vi "visObs (SubVI).vi"(1 "obsts":cluster{"x prior ":i32, "y prior":i32}[](array[cluster])) -> (0 "invisObsts":T1(array[cluster]))   [LabVIEW 2011]
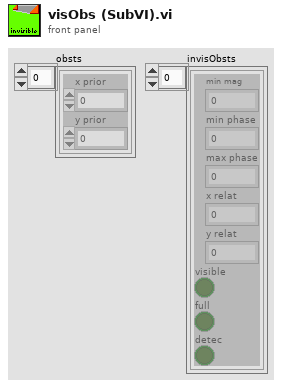
[diagram p1: front panel]
types:
  T1 = cluster{"min mag":dbl, "min phase":dbl, "max phase":dbl, "x relat":i32, "y relat":i32, "visible":bool, "full":bool, "detec":bool}[]
  T2 = cluster{"min mag":dbl, "min phase":dbl, "max phase":dbl, "x relat":i32, "y relat":i32, "visible":bool, "full":bool, "detec":bool}
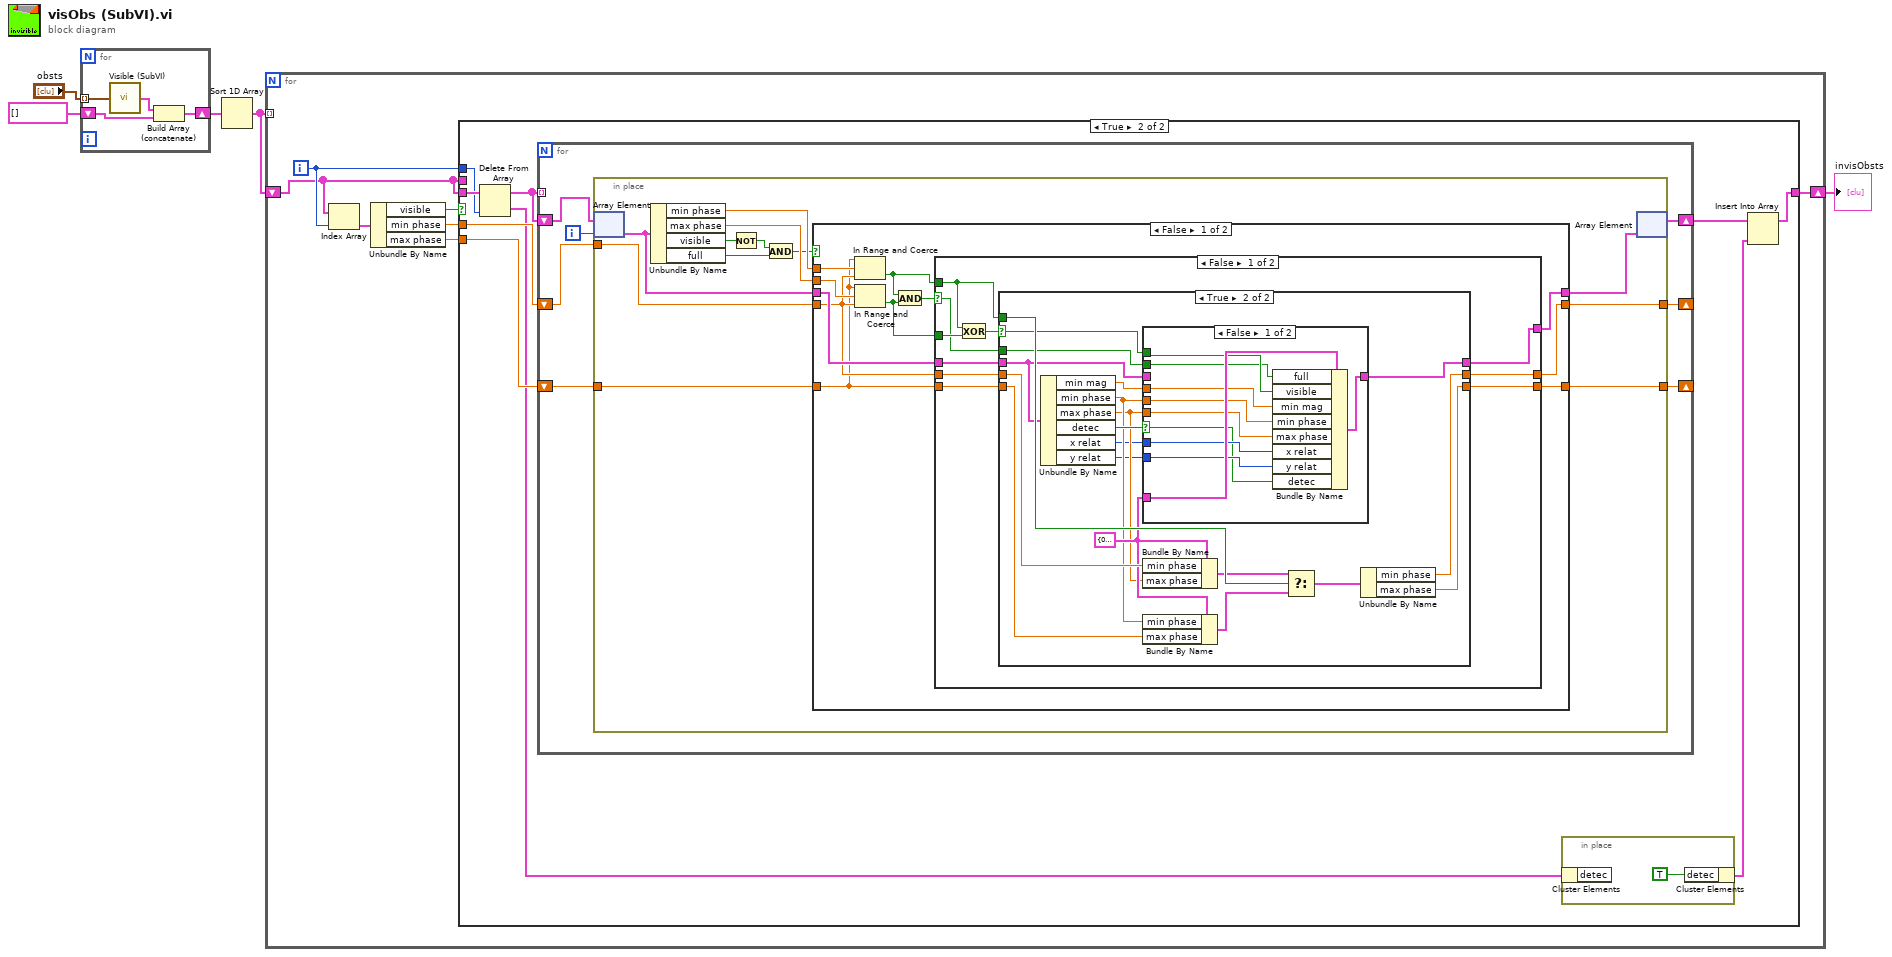
[diagram p0: block diagram]
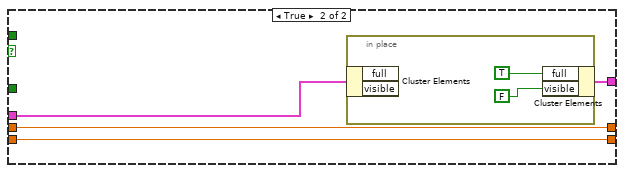
[diagram p5: hidden frame]
diagram:
  n1 = for {
    tunnel: "obsts" -> [w9] mode=indexing
    shift-right: [w8] -> w5
    shift-left: T1 [] -> [w7]
    n2 = call "Visible (SubVI).vi"("relatCoord"=w9) -> ("output cluster"=w6:T2)
    n3 = Build Array (concatenate)(w6, w7) -> (w8:T1)
  }
  n4 = Sort 1D Array(array=w5) -> (sorted array=w2:T1)
  n5 = for {
    shift-right: [w12] -> w1
    shift-left: w2 -> [w10]
    tunnel: w2 -> [_] mode=indexing
    i -> [w11]
    n6 = Index Array(array=w10, index=w11) -> (element=w16:T2)
    n7 = Unbundle By Name(w16) -> ("visible"=w13:bool, "min phase"=w15:dbl, "max phase"=w14:dbl)
    n8 = case shown="True" w13 {
      tunnel: w15 -> [_ w26]
      tunnel: w14 -> [_ w25]
      tunnel: w10 -> [_ _]
      tunnel: w10 -> [w17 w24]
      tunnel: [w17 w22] -> w12
      tunnel: w11 -> [_ w19]
      frame False {
      }
      frame True {
        n9 = Delete From Array(array=w24, index=w19) -> (deleted portion=w20:T2, array with subset deleted=w18:T1)  [unwired: 1 in]
        n10 = for {
          shift-right: [w34] -> w23
          shift-left: w18 -> [w33]
          shift-right: [w30] -> _
          shift-left: w26 -> [w32]
          shift-right: [w29] -> _
          shift-left: w25 -> [w31]
          tunnel: w18 -> [_] mode=indexing
          i -> [w28]
          n11 = in-place {
            in-place-border: w32 -> [w42]
            in-place-border: w31 -> [w41]
            in-place-border: [w40] -> w30
            in-place-border: [w39] -> w29
            n12 = in-place-array #1(w33, w28) -> (w44:T2)
            n13 = Unbundle By Name(w44) -> ("min phase"=w46:dbl, "max phase"=w45:dbl, "visible"=w38:bool, "full"=w35:bool)
            n14 = Not(x=w38) -> (.not. x?=w36:bool)
            n15 = And(x=w36, y=w35) -> (x .and. y?=w37:bool)
            n16 = case shown="False" w37 {
              tunnel: w46 -> [w56 _]
              tunnel: w45 -> [w55 _]
              tunnel: w44 -> [w54 w109]
              tunnel: [w53 w109] -> w43
              tunnel: w42 -> [w50 w107]
              tunnel: w41 -> [w49 w108]
              tunnel: [w48 w107] -> w40
              tunnel: [w47 w108] -> w39
              frame False {
                n17 = In Range and Coerce(upper limit=w49, x=w56, lower limit=w50) -> (In Range?=w52:bool)  [unwired: 1 out]
                n18 = In Range and Coerce(upper limit=w49, x=w55, lower limit=w50) -> (In Range?=w51:bool)  [unwired: 1 out]
                n19 = And(x=w52, y=w51) -> (x .and. y?=w57:bool)
                n20 = case shown="False" w57 {
                  selector: w57 -> [w58 _]
                  tunnel: [w61 w104] -> w53
                  tunnel: w54 -> [w64 w103]
                  tunnel: w52 -> [w66 _]
                  tunnel: w51 -> [w65 _]
                  tunnel: w50 -> [w63 w102]
                  tunnel: w49 -> [w62 w101]
                  tunnel: [w60 w102] -> w48
                  tunnel: [w59 w101] -> w47
                  frame False {
                    n21 = Exclusive Or(1:w65, 2:w66) -> (0:w67:bool)
                    n22 = case shown="True" w67 {
                      selector: w67 -> [_ w80]
                      tunnel: w66 -> [_ w89]
                      tunnel: w64 -> [w70 w76]
                      tunnel: w63 -> [w69 w88]
                      tunnel: w62 -> [w68 w86]
                      tunnel: [w70 w79] -> w61
                      tunnel: [w69 w84] -> w60
                      tunnel: [w68 w83] -> w59
                      tunnel: w58 -> [_ w78]
                      frame False {
                      }
                      frame True {
                        w81 = T2 {"min mag"=0.0, "min phase"=0.0, "max phase"=0.0, "x relat"=0, "y relat"=0, "visible"=TRUE, "full"=TRUE, "detec"=TRUE} ("input cluster")
                        n23 = Unbundle By Name(w76) -> ("min mag"=w75:dbl, "min phase"=w74:dbl, "max phase"=w73:dbl, "detec"=w77:bool, "x relat"=w72:i32, "y relat"=w71:i32)
                        n24 = case shown="False" w77 {
                          selector: w77 -> [w90 _]
                          tunnel: w81 -> [w99 _]
                          tunnel: w80 -> [w98 _]
                          tunnel: [w97 w100] -> w79
                          tunnel: w78 -> [w96 _]
                          tunnel: w76 -> [_ w100]
                          tunnel: w75 -> [w95 _]
                          tunnel: w74 -> [w94 _]
                          tunnel: w73 -> [w93 _]
                          tunnel: w72 -> [w92 _]
                          tunnel: w71 -> [w91 _]
                          frame False {
                            n25 = Bundle By Name(cluster=w99, "full"=w96, "visible"=w98, "min mag"=w95, "min phase"=w94, "max phase"=w93, "x relat"=w92, "y relat"=w91, "detec"=w90) -> (w97:T2)
                          }
                          frame True {
                          }
                        }
                        n26 = Bundle By Name(cluster=w81, "min phase"=w88, "max phase"=w73) -> (w87:T2)
                        n27 = Bundle By Name(cluster=w81, "min phase"=w74, "max phase"=w86) -> (w85:T2)
                        n28 = Select(t=w87, s=w89, f=w85) -> (s? t:f=w82:T2)
                        n29 = Unbundle By Name(w82) -> ("min phase"=w84:dbl, "max phase"=w83:dbl)
                      }
                    }
                  }
                  frame True {
                    n30 = in-place {
                      n31 = in-place-cluster #2(w103) -> ()  [unwired: 2 out]
                      n32 = in-place-cluster #2("full"=TRUE, "visible"=FALSE) -> (w104:T2)
                    }
                  }
                }
              }
              frame True {
              }
            }
            n33 = in-place-array #1(w43) -> (w34:T1)  [unwired: 1 out]
          }
        }
        n34 = in-place {
          n35 = in-place-cluster #3(w20) -> ()  [unwired: 1 out]
          n36 = in-place-cluster #3("detec"=TRUE) -> (w21:T2)
        }
        n37 = Insert Into Array(array=w23, new element=w21) -> (w22:T1)  [unwired: 1 in]
      }
    }
  }
  "invisObsts" <- w1
